vi "Event Handler.vi"(0 "uService Test in":refnum<class "test_us.lvclass">, 5 "Event type":T1, 7 "Item Name":string, 9 "Data":variant, 11 "error in (no error)":errorcluster) -> (4 "uService Test out":refnum<class "test_us.lvclass">, 15 "error out":errorcluster)   [LabVIEW 2026, in "test_us.lvlib" / "test_us.lvclass"]
uses:
  test_us.lvclass
  C:/LabVIEW Code/TALOS/talos/Father of all uServices/Father of all uServices/Father of all uServices.lvclass
  C:/LabVIEW Code/TALOS/builds/Actor Framework PPL/Actor Framework.lvlibp/1abvi3w/vi.lib/ActorFramework/Actor/Actor.lvclass
  Father of all uServices/Father of all uServices/Event Handler Items.ctl
  Guardian/Guardian Messages/Message to uService Msg/Message to uService Msg.lvclass/Message to uService Msg.ctl
  Ancestor/Ancestor/Ancestor.lvclass/Ancestor.ctl
  Guardian/Guardian Messages/TCP-SV Message Interpreter Msg/TCP-SV Message Interpreter Msg.lvclass/TCP-SV Message Interpreter Msg.ctl
  Classes/Circus Shared Variables/Circus Shared Variables.lvclass/Circus Shared Variables.ctl
  Test uS Consumer case selector.ctl
  Father of all uServices/Father of all uServices/Father of all uServices.lvclass/Father of all uServices.ctl
  Father of all uServices/Father of all uServices Messages/Consumer Msg/Consumer Msg.lvclass/Consumer Msg.ctl
  Guardian/Guardian/Requests.ctl
  Guardian/Guardian Messages/Requests from uServices Msg/Requests from uServices Msg.lvclass/Requests from uServices Msg.ctl
  test_us.lvclass/test_us.ctl
  Guardian/Guardian Messages/Message to uService Msg/Send Message to uService.vi
  Support VIs/Substitute Error.vi
  Ancestor/Ancestor/Read ID.vi
  Father of all uServices/Father of all uServices Messages/Consumer Msg/Send Consumer.vi
  Guardian/Guardian Messages/Requests from uServices Msg/Send Requests from uServices.vi
  Support VIs/Generate Error.vi
  FGV/Error Memory/Get Error Description.vi
  Support VIs/Get PC name.vi
  Support VIs/Get Class Name.vi
  <vilib>/Utility/error.llb/Clear Errors.vi
  FGV/Error Memory/Error Memory Core.vi
  <vilib>/AdvancedString/Delimited String to 1D String Array.vi
  <vilib>/AdvancedString/Delimited String to 1D String Array (string).vi
  Support VIs/Circus Root Path.vi
  FGV/Error Memory/Error Crt Lvl checker.vi
  FGV/Error Memory/Error Memory Core.vi/40c8088d-b597-4017-91af-faa98e00292e.vi
  FGV/Error Memory/Error Memory Core.vi/d4a3ab98-063c-4e44-b43d-fbdcfe6c2be2.vi
  Father of all uServices/Father of all uServices/Father of all uServices.lvclass
  C:/LabVIEW Code/TALOS/talos/Ancestor/Ancestor/Ancestor.lvclass
  builds/Actor Framework PPL/Actor Framework.lvlibp/1abvi3w/vi.lib/ActorFramework/Message Enqueuer/Enqueue.vi
  Support VIs/Global Memory.vi
  <vilib>/Utility/LVClass/Get LV Class Name.vi
  Support VIs/Is in Packed Library.vi
  Support VIs/TALOS Root path.vi
  Support VIs/Read CSV worksheet.vi
  Support VIs/Global Constants.vi
  <vilib>/Utility/error.llb/General Error Handler.vi
  Support VIs/Error Log.vi
  builds/Actor Framework PPL/Actor Framework.lvlibp/1abvi3w/vi.lib/ActorFramework/Actor/Read Self Enqueuer.vi
  <userlib>/_OpenG.lib/lvdata/lvdata.llb/Get Strings from Enum__ogtk.vi
  Father of all uServices/Father of all uServices/Children Methods/Get GUI Item Ref.vi
  Guardian/Guardian Messages/Message to uService Msg/Message to uService Msg.lvclass
  Ancestor/Ancestor/Ancestor.lvclass
  <vilib>/Comparison/Equal/Equal Functor/Equal Functor.lvclass
  Guardian/Guardian Messages/TCP-SV Message Interpreter Msg/TCP-SV Message Interpreter Msg.lvclass
  Father of all uServices/Father of all uServices Messages/Consumer Msg/Consumer Msg.lvclass
  Guardian/Guardian Messages/Requests from uServices Msg/Requests from uServices Msg.lvclass
  Guardian/Guardian Messages/I Exist Msg/I Exist Msg.lvclass
  Classes/Circus Shared Variables/Circus Shared Variables.lvclass
  builds/Actor Framework PPL/Actor Framework.lvlibp/1abvi3w/vi.lib/ActorFramework/Actor/Actor.lvclass
  Classes/Error Filter/Error Filter.lvclass
  Guardian/Guardian/Guardian.lvclass
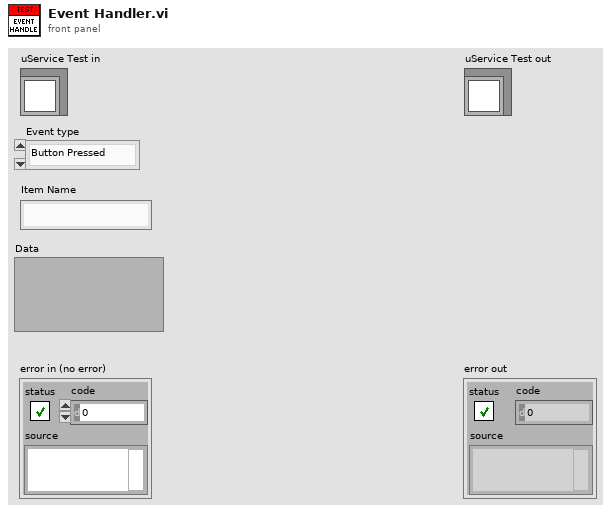
[diagram p1: front panel]
types:
  T1 = typedef "TALOS.lvlib/Father of all uServices.lvlib/Father of all uServices.lvclass/Event Handler Items.ctl" = enum16{"Button Pressed", "Message", "Ready to launch?", "Safe Mode", "Start RUN", "Stop RUN"}
  T2 = typedef "test_us.lvlib/test_us.lvclass/Test uS Consumer case selector.ctl" = enum16{"graph", "infinite", "Start infinite", "Check infinite", "Stop infinite", "Delayed message"}
  T3 = typedef "TALOS.lvlib/Guardian.lvlib/Guardian.lvclass/Requests.ctl" = enum16{"Ready to Launch", "Start RUN", "Stop RUN", "Update DAQ Params", "Update Error Listbox", "Update Run Status", "Update Kasli Log", "Run Stopped with Errors", "Switch uS View", "Dismiss All Errors"}
  T4 = cluster{"ID":string, "Alive":bool, "Last Seen":timestamp}
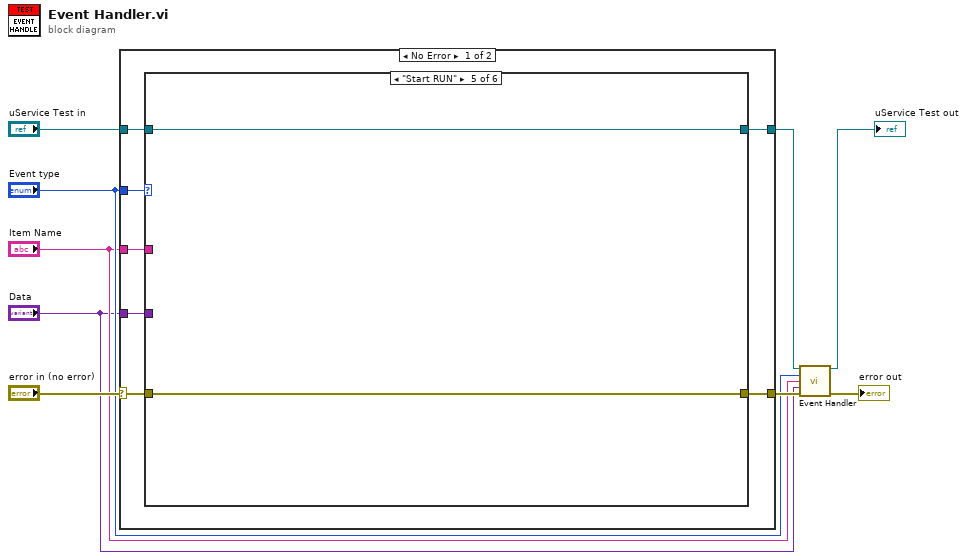
[diagram p0: block diagram]
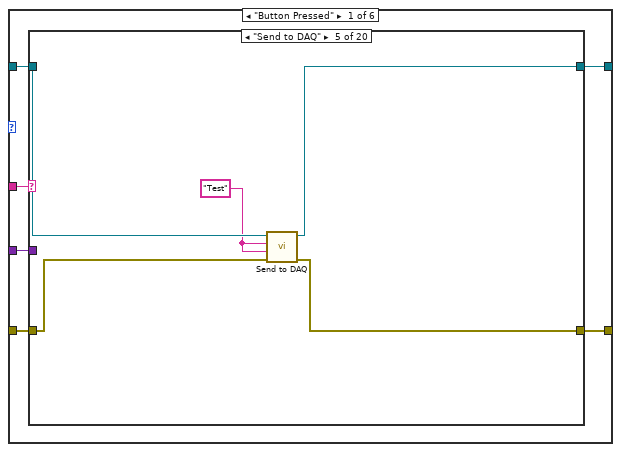
[diagram p2: hidden frame]
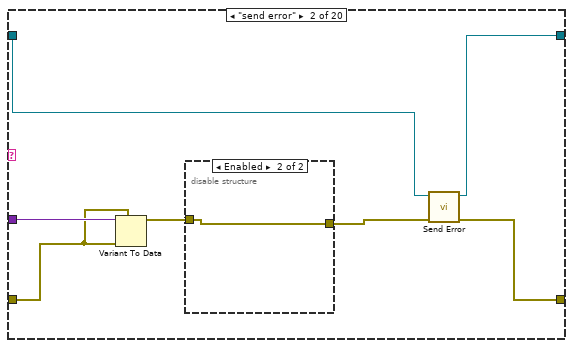
[diagram p4: hidden frame]
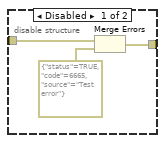
[diagram p5: hidden frame]
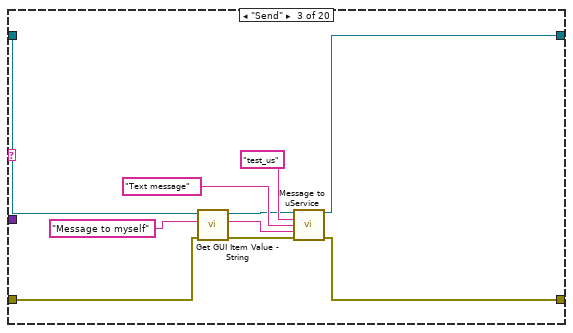
[diagram p6: hidden frame]
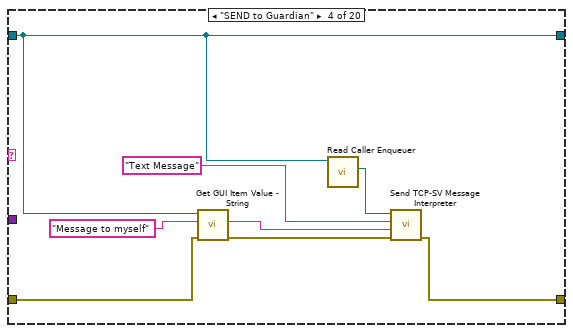
[diagram p7: hidden frame]
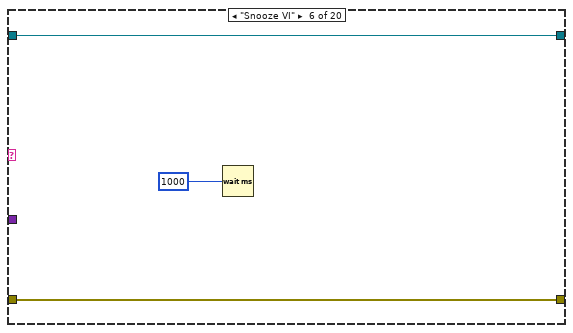
[diagram p8: hidden frame]
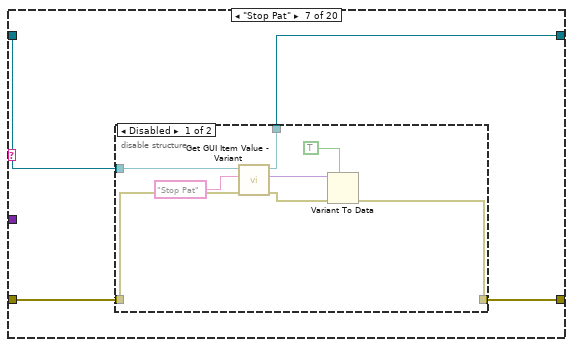
[diagram p9: hidden frame]
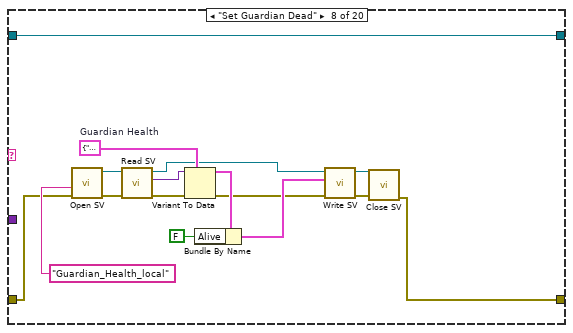
[diagram p11: hidden frame]
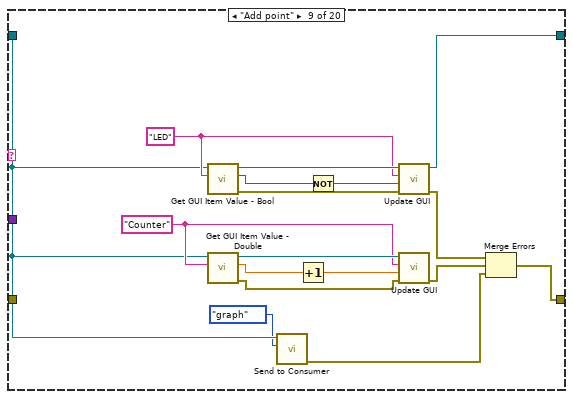
[diagram p12: hidden frame]
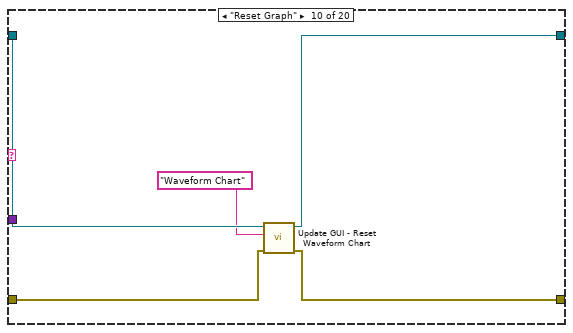
[diagram p13: hidden frame]
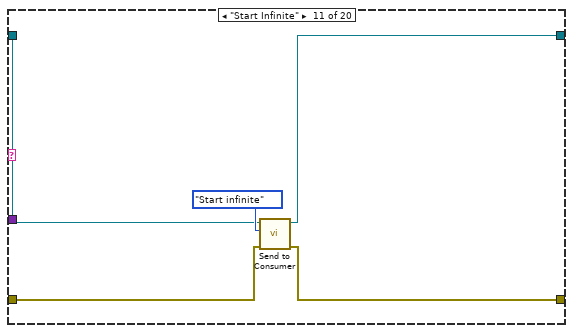
[diagram p14: hidden frame]
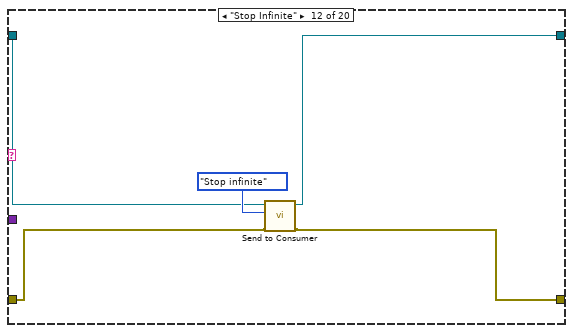
[diagram p15: hidden frame]
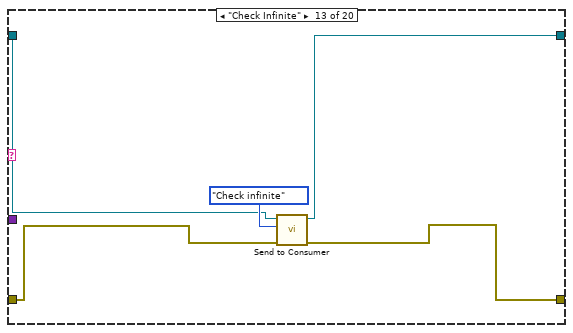
[diagram p16: hidden frame]
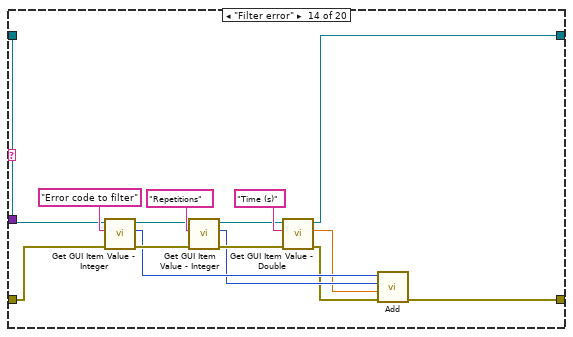
[diagram p17: hidden frame]
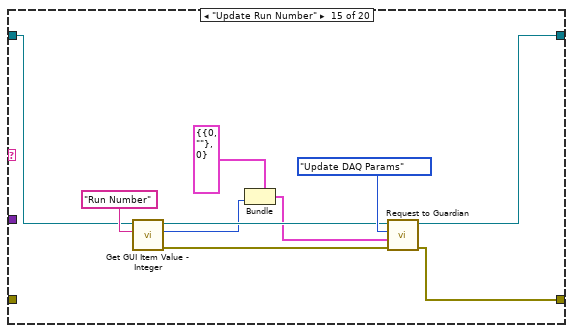
[diagram p18: hidden frame]
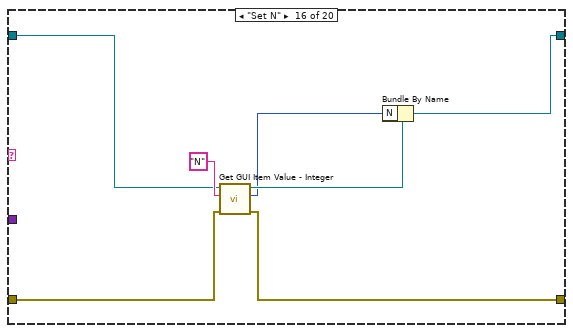
[diagram p19: hidden frame]
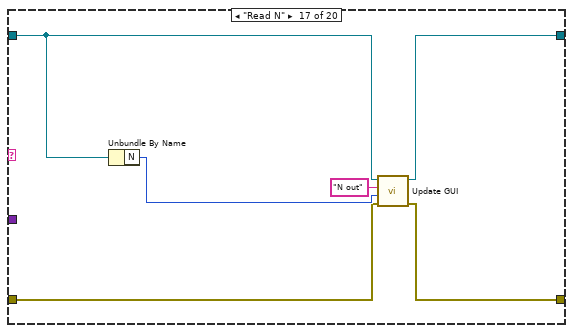
[diagram p20: hidden frame]
diagram:
  n1 = case shown="No Error" "error in (no error)" {
    selector: "error in (no error)" -> [w14 w226]
    tunnel: [w15 w226] -> w7
    tunnel: [w10 w225] -> w5
    tunnel: "uService Test in" -> [w13 w225]
    tunnel: "Event type" -> [w16 _]
    tunnel: "Item Name" -> [w12 _]
    tunnel: "Data" -> [w11 _]
    frame No Error {
      n2 = case shown="\"Start RUN\"" w16 {
        tunnel: [w22 w191 w194 w199 w222 w224] -> w15
        tunnel: w14 -> [w19 w191 w193 w203 w222 w224]
        tunnel: w12 -> [w20 _ _ w202 _ _]
        tunnel: w13 -> [w21 w190 w197 w200 w221 w223]
        tunnel: w11 -> [w18 _ _ w201 _ _]
        tunnel: [w17 w190 w192 w198 w221 w223] -> w10
        frame "Button Pressed" {
          n3 = case shown="\"Send to DAQ\"" w20 {
            tunnel: w19 -> [w24 w30 w41 w52 w58 w60 w63 w90 _ w111 w116 w121 w126 w135 _ w155 w162 w168 w183 w187]
            tunnel: [w24 w27 w38 w47 w57 w60 w64 w85 w96 w110 w115 w120 w125 w130 w148 w154 w161 w167 w176 w186] -> w22
            tunnel: w21 -> [w23 w29 w43 w46 w56 w59 w65 w76 w95 w113 w117 w122 w127 w138 w152 w159 w164 w172 w175 w189]
            tunnel: w18 -> [_ w31 _ _ _ _ _ _ _ _ _ _ _ _ _ _ _ _ w184 _]
            tunnel: [w23 w25 w36 w46 w55 w59 w62 w76 w92 w109 w114 w119 w124 w129 w144 w156 w165 w171 w174 w189] -> w17
            frame Default {
            }
            frame "send error" {
              n4 = Variant To Data(error in=w30, type=w30, Variant=w31) -> (data=w28:errorcluster)  [unwired: 1 out]
              n5 = disable-structure shown="Enabled" {
                disable-tunnel: w28 -> [w34 w35]
                disable-tunnel: [w33 w35] -> w26
                frame Disabled {
                  n6 = Merge Errors(w34, errorcluster {"status"=TRUE, "code"=6665, "source"="Test error"} ("error in")) -> (w33:errorcluster)
                }
                frame Enabled {
                }
              }
              n7 = call-dynamic "Send Error.vi"("error in (no error)"=w26, "Father of all uServices in"=w29) -> ("error out"=w27:errorcluster, "Father of all uServices out"=w25:refnum<class "test_us.lvclass">)  [unwired: 8 in]
            }
            frame "Send" {
              n8 = call "Get GUI Item Value - String.vi"("error in (no error)"=w41, "FP Item Name"="Message to myself", "uService Template in"=w43) -> ("error out"=w40:errorcluster, "Value"=w39:string, "uService Template out"=w37:refnum<class "test_us.lvclass">)  [unwired: 6 in]
              n9 = call "Message to uService.vi"("Father of all uServices in"=w37, "uService ID"="test_us", "Message"="Text message", "Data"=w39, "error in (no error)"=w40) -> ("Father of all uServices out"=w36:refnum<class "test_us.lvclass">, "error out"=w38:errorcluster)  [unwired: 9 in]
            }
            frame "SEND to Guardian" {
              n10 = call "Get GUI Item Value - String.vi"("error in (no error)"=w52, "FP Item Name"="Message to myself", "uService Template in"=w46) -> ("error out"=w48:errorcluster, "Value"=w49:string)  [unwired: 6 in, 1 out]
              n11 = call "Read Caller Enqueuer.vi"("Actor"=w46) -> ("Caller Enqueuer"=w51:refnum<class "Message Enqueuer.lvclass">)  [unwired: 10 in]
              n12 = call "Send TCP-SV Message Interpreter.vi"("error in (no error)"=w48, "Data"=w49, "Message"="Text Message", "Message Enqueuer"=w51) -> ("error out"=w47:errorcluster)  [unwired: 6 in, 1 out]
            }
            frame "Send to DAQ" {
              w54 = "Test" ("Data Name")
              n13 = call "Send to DAQ.vi"("error in (no error)"=w58, "Data"=w54, "Data Name"=w54, "Father of all uServices in"=w56) -> ("error out"=w57:errorcluster, "Father of all uServices out"=w55:refnum<class "test_us.lvclass">)  [unwired: 6 in]
            }
            frame "Snooze VI" {
              n14 = Wait (ms)(milliseconds to wait=u32 1000) -> ()  [unwired: 1 out]
            }
            frame "Stop Pat" {
              n15 = disable-structure shown="Disabled" {
                disable-tunnel: w65 -> [w70 w74]
                disable-tunnel: [w68 w75] -> w64
                disable-tunnel: w63 -> [w67 w75]
                disable-tunnel: [w66 w74] -> w62
                frame Disabled {
                  n16 = call "Get GUI Item Value - Variant.vi"("error in (no error)"=w67, "FP Item Name"="Stop Pat", "uService Template in"=w70) -> ("error out"=w71:errorcluster, "Value"=w72:variant, "uService Template out"=w66:refnum<class "test_us.lvclass">)  [unwired: 6 in]
                  n17 = Variant To Data(error in=w71, type=TRUE, Variant=w72) -> (error out=w68:errorcluster)  [unwired: 1 out]
                }
                frame Enabled {
                }
              }
            }
            frame "Set Guardian Dead" {
              w80 = T4 {"ID"="", "Alive"=FALSE, "Last Seen"=timestamp(0 s since 1904-01-01)}  # Guardian Health
              n18 = call "Open SV.vi"("error in (no error)"=w90, "SV Name"="Guardian_Health_local") -> ("error out"=w84:errorcluster, "AEgIS Shared Variables out"=w83:refnum<class "Circus Shared Variables.lvclass">)  [unwired: 8 in]
              n19 = call "Read SV.vi"("error in (no error)"=w84, "AEgIS Shared Variables in"=w83) -> ("error out"=w82:errorcluster, "Variant"=w81:variant, "AEgIS Shared Variables out"=w77:refnum<class "Circus Shared Variables.lvclass">)  [unwired: 7 in]
              n20 = Variant To Data(error in=w82, type=w80, Variant=w81) -> (data=w79:T4, error out=w78:errorcluster)
              n21 = Bundle By Name(cluster=w79, "Alive"=FALSE) -> (w88:T4)
              n22 = call "Write SV.vi"("error in (no error)"=w78, "Variant"=w88, "AEgIS Shared Variables in"=w77) -> ("error out"=w87:errorcluster, "AEgIS Shared Variables out"=w86:refnum<class "Circus Shared Variables.lvclass">)  [unwired: 7 in]
              n23 = call "Close SV.vi"("error in (no error)"=w87, "AEgIS Shared Variables in"=w86) -> ("error out"=w85:errorcluster)  [unwired: 7 in, 2 out]
            }
            frame "Add point" {
              w102 = "Counter" ("GUI Item Name")
              w106 = "LED" ("GUI Item Name")
              n24 = call "Get GUI Item Value - Bool.vi"("FP Item Name"=w106, "uService Template in"=w95) -> ("error out"=w107:errorcluster, "Value"=w105:bool, "uService Template out"=w108:refnum<class "test_us.lvclass">)  [unwired: 7 in]
              n25 = call "Get GUI Item Value - Double.vi"("FP Item Name"=w102, "uService Template in"=w95) -> ("error out"=w99:errorcluster, "Value"=w101:dbl, "uService Template out"=w103:refnum<class "test_us.lvclass">)  [unwired: 7 in]
              n26 = call "Send to Consumer.vi"("Case ID"=Test_uS_Consumer_case_selector."graph" ("arsnars consumer case selector"), "uService Template in"=w95) -> ("error out"=w94:errorcluster)  [unwired: 8 in, 1 out]
              n27 = Increment(x=w101) -> (x+1=w100:dbl)
              n28 = Not(x=w105) -> (.not. x?=w104:bool)
              n29 = call "Update GUI.vi"("error in (no error)"=w107, "Data"=w104, "GUI Item Name"=w106, "uService Template in"=w108) -> ("error out"=w98:errorcluster, "uService Template out"=w92:refnum<class "test_us.lvclass">)  [unwired: 6 in]
              n30 = call "Update GUI.vi"("error in (no error)"=w99, "Data"=w100, "GUI Item Name"=w102, "uService Template in"=w103) -> ("error out"=w97:errorcluster)  [unwired: 6 in, 1 out]
              n31 = Merge Errors(w98, w97, w94) -> (w96:errorcluster)
            }
            frame "Reset Graph" {
              n32 = call "Update GUI - Reset Waveform Chart.vi"("error in (no error)"=w111, "GUI Item Name"="Waveform Chart", "uService Template in"=w113) -> ("error out"=w110:errorcluster, "uService Template out"=w109:refnum<class "test_us.lvclass">)  [unwired: 7 in]
            }
            frame "Start Infinite" {
              n33 = call "Send to Consumer.vi"("error in (no error)"=w116, "Case ID"=Test_uS_Consumer_case_selector."Start infinite" ("arsnars consumer case selector"), "uService Template in"=w117) -> ("error out"=w115:errorcluster, "uService Template out"=w114:refnum<class "test_us.lvclass">)  [unwired: 7 in]
            }
            frame "Stop Infinite" {
              n34 = call "Send to Consumer.vi"("error in (no error)"=w121, "Case ID"=Test_uS_Consumer_case_selector."Stop infinite" ("arsnars consumer case selector"), "uService Template in"=w122) -> ("error out"=w120:errorcluster, "uService Template out"=w119:refnum<class "test_us.lvclass">)  [unwired: 7 in]
            }
            frame "Check Infinite" {
              n35 = call "Send to Consumer.vi"("error in (no error)"=w126, "Case ID"=Test_uS_Consumer_case_selector."Check infinite" ("arsnars consumer case selector"), "uService Template in"=w127) -> ("error out"=w125:errorcluster, "uService Template out"=w124:refnum<class "test_us.lvclass">)  [unwired: 7 in]
            }
            frame "Filter error" {
              n36 = call "Get GUI Item Value - Integer.vi"("error in (no error)"=w135, "FP Item Name"="Error code to filter", "uService Template in"=w138) -> ("error out"=w141:errorcluster, "Value"=w134:i32, "uService Template out"=w137:refnum<class "test_us.lvclass">)  [unwired: 6 in]
              n37 = call "Get GUI Item Value - Integer.vi"("error in (no error)"=w141, "FP Item Name"="Repetitions", "uService Template in"=w137) -> ("error out"=w140:errorcluster, "Value"=w133:i32, "uService Template out"=w136:refnum<class "test_us.lvclass">)  [unwired: 6 in]
              n38 = call "Get GUI Item Value - Double.vi"("error in (no error)"=w140, "FP Item Name"="Time (s)", "uService Template in"=w136) -> ("error out"=w131:errorcluster, "Value"=w132:dbl, "uService Template out"=w129:refnum<class "test_us.lvclass">)  [unwired: 6 in]
              n39 = call "Add.vi"("error in (no error)"=w131, "Time (s)"=w132, "Repetitions"=w133, "Error Code"=w134) -> ("error out"=w130:errorcluster)  [unwired: 7 in]
            }
            frame "Update Run Number" {
              n40 = call "Get GUI Item Value - Integer.vi"("FP Item Name"="Run Number", "uService Template in"=w152) -> ("error out"=w150:errorcluster, "Value"=w146:i32, "uService Template out"=w149:refnum<class "test_us.lvclass">)  [unwired: 7 in]
              n41 = Bundle(cluster=cluster{cluster{u16, string}, i32} {{0, ""}, 0}, w146) -> (w145:cluster{cluster{u16, string}, i32})  [unwired: 1 in]
              n42 = call "Request to Guardian.vi"("error in (no error)"=w150, "Data"=w145, "Requests"=Requests."Update DAQ Params", "Father of all uServices in"=w149) -> ("error out"=w148:errorcluster, "Father of all uServices out"=w144:refnum<class "test_us.lvclass">)  [unwired: 6 in]
            }
            frame "Set N" {
              n43 = call "Get GUI Item Value - Integer.vi"("error in (no error)"=w155, "FP Item Name"="N", "uService Template in"=w159) -> ("error out"=w154:errorcluster, "Value"=w157:i32, "uService Template out"=w158:refnum<class "test_us.lvclass">)  [unwired: 6 in]
              n44 = Bundle By Name(cluster=w158, "N"=w157) -> (w156:refnum<class "test_us.lvclass">)
            }
            frame "Read N" {
              n45 = Unbundle By Name(w164) -> ("N"=w163:i32)
              n46 = call "Update GUI.vi"("error in (no error)"=w162, "Data"=w163, "GUI Item Name"="N out", "uService Template in"=w164) -> ("error out"=w161:errorcluster, "uService Template out"=w165:refnum<class "test_us.lvclass">)  [unwired: 6 in]
            }
            frame "Switch uS View" {
              n47 = call "Request to Guardian.vi"("error in (no error)"=w168, "Data"="Error Manager", "Requests"=Requests."Switch uS View", "Father of all uServices in"=w172) -> ("error out"=w167:errorcluster, "Father of all uServices out"=w171:refnum<class "test_us.lvclass">)  [unwired: 6 in]
            }
            frame "Delayed message" {
              n48 = Variant To Data(error in=w183, type=0.0, Variant=w184) -> (data=w180:dbl, error out=w182:errorcluster)
              n49 = call "Delayed Send to Consumer.vi"("Seconds (5)"=w180, "error in (no error)"=w182, "Case ID"=Test_uS_Consumer_case_selector."Delayed message" ("arsnars consumer case selector"), "Father of all uServices in"=w175) -> ("error out"=w185:errorcluster, "Father of all uServices out"=w173:refnum<class "test_us.lvclass">)  [unwired: 6 in]
              n50 = Get Date/Time In Seconds() -> (seconds since 1Jan1904=w177:timestamp)
              n51 = call "Update GUI.vi"("error in (no error)"=w185, "Data"=w177, "GUI Item Name"="Delay submit time", "uService Template in"=w173) -> ("error out"=w176:errorcluster, "uService Template out"=w174:refnum<class "test_us.lvclass">)  [unwired: 6 in]
            }
            frame "Send I exist" {
              n52 = call "Read Caller Enqueuer.vi"("Actor"=w189) -> ("Caller Enqueuer"=w188:refnum<class "Message Enqueuer.lvclass">)  [unwired: 10 in]
              n53 = call "Send I Exist.vi"("error in (no error)"=w187, "Message Enqueuer"=w188) -> ("error out"=w186:errorcluster)  [unwired: 8 in, 1 out]
            }
          }
        }
        frame "Ready to launch?" {
        }
        frame "Safe Mode" {
          n54 = call "Update GUI.vi"("error in (no error)"=w193, "Data"=TRUE, "GUI Item Name"="Safe Mode", "uService Template in"=w197) -> ("error out"=w194:errorcluster, "uService Template out"=w192:refnum<class "test_us.lvclass">)  [unwired: 6 in]
        }
        frame "Message" {
          n55 = case shown="Default" w202 {
            selector: w202 -> [_ w212 w216]
            tunnel: w203 -> [w205 w213 w217]
            tunnel: w201 -> [_ w214 _]
            tunnel: w200 -> [w204 w207 w218]
            tunnel: [w205 w211 w220] -> w199
            tunnel: [w204 w206 w215] -> w198
            frame Default {
            }
            frame "Text message" {
              n56 = Variant To Data(error in=w213, type=w212, Variant=w214) -> (data=w209:string, error out=w210:errorcluster)
              n57 = call "Update GUI.vi"("error in (no error)"=w210, "Data"=w209, "GUI Item Name"="Message Received", "uService Template in"=w207) -> ("error out"=w211:errorcluster, "uService Template out"=w206:refnum<class "test_us.lvclass">)  [unwired: 6 in]
            }
            frame "Broadcast_message" {
              n58 = call "Update GUI.vi"("error in (no error)"=w217, "Data"=w216, "GUI Item Name"="Message Received", "uService Template in"=w218) -> ("error out"=w220:errorcluster, "uService Template out"=w215:refnum<class "test_us.lvclass">)  [unwired: 6 in]
            }
          }
        }
        frame "Start RUN" {
        }
        frame "Stop RUN" {
        }
      }
    }
    frame Error {
    }
  }
  n59 = call-parent "Event Handler.vi"("uService Template in"=w5, "Event type"="Event type", "Item Name"="Item Name", "Data"="Data", "error in (no error)"=w7) -> ("uService Template out"=→"uService Test out":refnum<class "test_us.lvclass">, "error out"=→"error out":errorcluster)  [unwired: 9 in]
